vi "Status - motion only.vi"(8 "error in (no error)":errorcluster, 11 "VISA resource name":refnum<visa-resource-name>) -> (0 "error out":errorcluster, 3 "VISA resource out":refnum<visa-resource-name>, 4 "Motion Stopped":bool, 5 "Limit Switch Activated":bool)   [LabVIEW 2017]
doc: "Read serial buffer during motion.\nParse response string for ^ or O characters.\n^ motion is complete\nO limit switch has been hit"
panel:
  out "Response String ('/' codes)":string
  in  "Timeout, s":dbl=0.5 format="%#_13g"
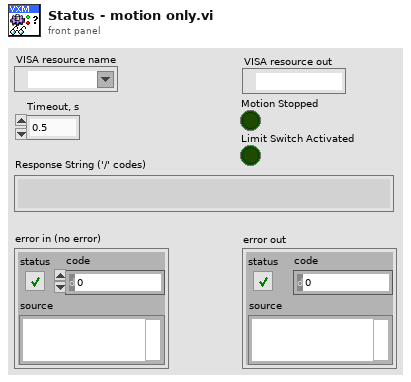
[diagram p1: front panel]
types:
  T1 = enum16{"Cmd-Response", "Write Only", "Read Only"}
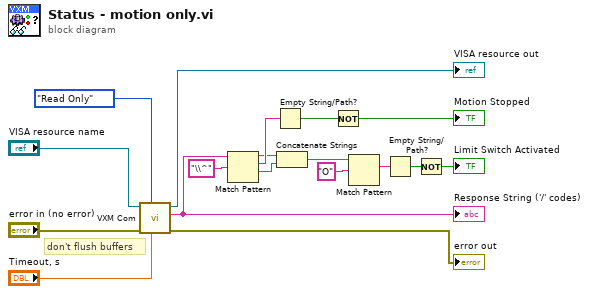
[diagram p0: block diagram]
diagram:
  # "don't flush buffers"
  n1 = call "VXM Com.vi"("Timeout, s"="Timeout, s", "Operation"=T1."Read Only", "error in (no error)"="error in (no error)", "VISA resource name"="VISA resource name") -> ("error out"=→"error out":errorcluster, "Response String ('/' codes)"=w5:string, "VISA resource out"=→"VISA resource out":refnum<visa-resource-name>)  [unwired: 5 in]
  "Response String ('/' codes)" <- w5
  n2 = Match Pattern(string=w5, regular expression="\\^") -> (before substring=w11:string, match substring=w13:string, after substring=w10:string)  [unwired: 1 in, 1 out]
  n3 = Empty String/Path?(string/path=w13) -> (empty?=w12:bool)
  n4 = Concatenate Strings(w11, w10) -> (w6:string)
  n5 = Not(x=w12) -> (.not. x?=→"Motion Stopped":bool)
  n6 = Match Pattern(string=w6, regular expression="O") -> (match substring=w8:string)  [unwired: 1 in, 3 out]
  n7 = Empty String/Path?(string/path=w8) -> (empty?=w9:bool)
  n8 = Not(x=w9) -> (.not. x?=→"Limit Switch Activated":bool)
